vi "Servo-Centerization.vi"(1 "HALF Cam angle constant":dbl, 2 "Cartez":dbl) -> (0 "Rounded Error":dbl)   [LabVIEW 2011]
panel:
  out "Error":dbl
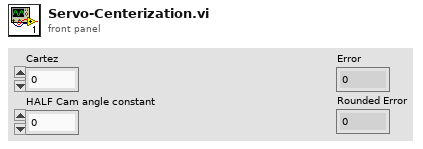
[diagram p1: front panel]
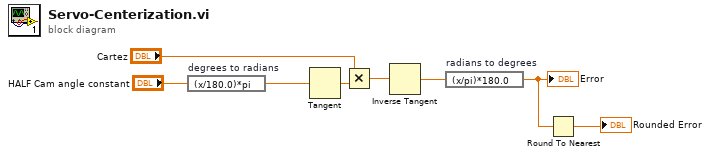
[diagram p0: block diagram]
diagram:
  n1 = expression code="(x/180.0)*pi" "degrees to radians"("HALF Cam angle constant") -> (w3:dbl)
  n2 = Tangent(1:w3) -> (0:w8:dbl)
  n3 = Multiply(x="Cartez", y=w8) -> (x*y=w5:dbl)
  n4 = Inverse Tangent(1:w5) -> (0:w6:dbl)
  n5 = expression code="(x/pi)*180.0" "radians to degrees"(w6) -> (w1:dbl)
  "Error" <- w1
  n6 = Round To Nearest(number=w1) -> (nearest integer value=→"Rounded Error":dbl)
